vi "get_line_scan_time.vi"(8 "error in (no error)":errorcluster, 11 "TrajectoryDL121017Hopping in":refnum<class "TrajectoryDL121017Hopping.lvclass">) -> (0 "error out":errorcluster, 2 "line scan time":dbl[unit], 3 "TrajectoryDL121017Hopping out":refnum<class "TrajectoryDL121017Hopping.lvclass">)   [LabVIEW 2010, in "TrajectoryDL121017Hopping.lvclass"]
uses:
  TrajectoryDL121017Hopping.lvclass
  TrajectoryDL121017Hopping.lvclass/TrajectoryDL121017Hopping.ctl
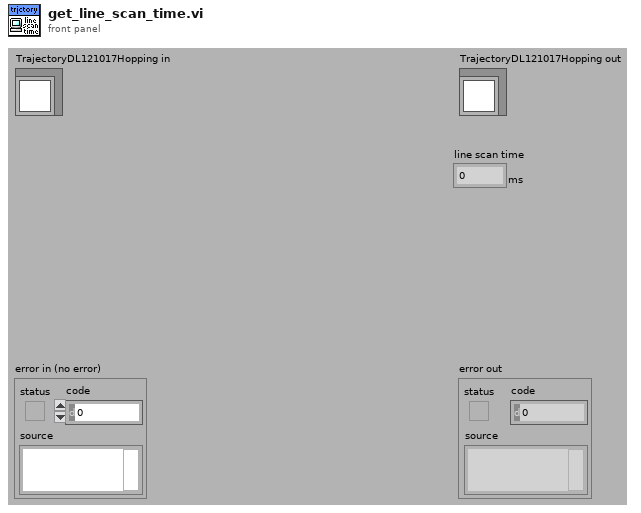
[diagram p1: front panel]
types:
  T1 = typedef "TrajectoryDL121017Hopping.lvclass/subpattern_type_enum.ctl" = enum16{"none", "spiral"}
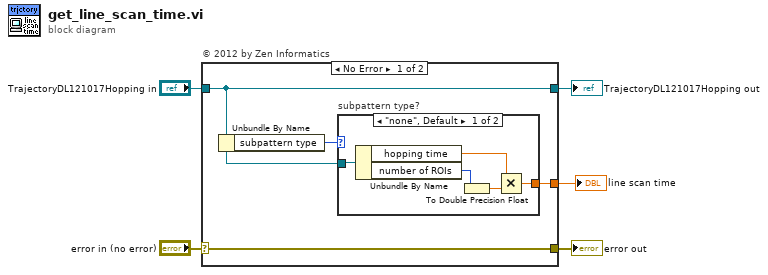
[diagram p0: block diagram]
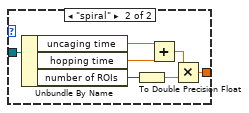
[diagram p2: hidden frame]
diagram:
  n1 = case "© 2012 by Zen Informatics" shown="No Error" "error in (no error)" {
    selector: "error in (no error)" -> [w9 w23]
    tunnel: [w9 w23] -> w4
    tunnel: [w7 w22] -> w2
    tunnel: "TrajectoryDL121017Hopping in" -> [w7 w22]
    tunnel: [w8 _] -> w1
    frame No Error {
      n2 = Unbundle By Name(w7) -> ("subpattern type"=w6:T1)
      n3 = case "subpattern type?" shown="\"none\", Default" w6 {
        tunnel: w7 -> [w14 w21]
        tunnel: [w11 w16] -> w8
        frame "none", Default {
          n4 = Unbundle By Name(w14) -> ("hopping time"=w13:dbl[unit], "number of ROIs"=w10:i32)
          n5 = To Double Precision Float(number=w10) -> (double precision float=w12:dbl)
          n6 = Multiply(x=w13, y=w12) -> (x*y=w11:dbl[unit])
        }
        frame "spiral" {
          n7 = Unbundle By Name(w21) -> ("uncaging time"=w19:dbl[unit], "hopping time"=w18:dbl[unit], "number of ROIs"=w15:i32)
          n8 = To Double Precision Float(number=w15) -> (double precision float=w20:dbl)
          n9 = Add(x=w19, y=w18) -> (x+y=w17:dbl[unit])
          n10 = Multiply(x=w17, y=w20) -> (x*y=w16:dbl[unit])
        }
      }
    }
    frame Error {
    }
  }
  "error out" <- w4
  "TrajectoryDL121017Hopping out" <- w2
  "line scan time" <- w1
